vi "9203 8Ch Analog Input.vi"(1 "9203 I/O":T1={"9203 AI0"="NI 9203/AI0", "9203 AI1"="NI 9203/AI1", "9203 AI2"="NI 9203/AI2", "9203 AI3"="NI 9203/AI3", "9203 AI4"="NI 9203/AI4", "9203 AI5"="NI 9203/AI5", "9203 AI6"="NI 9203/AI6", "9203 AI7"="NI 9203/AI7"}) -> (0 "Packets":u64[](array[numeric]))   [LabVIEW 2010]
uses:
  <vilib>/eio/EIONode/EIONode.xnode
  <vilib>/rvi/eio/nirviEIOImplementation/nirviEIOImplementation.xnode
  <vilib>/rvi/eio/common/nirviEmuClasses.ctl
  <vilib>/rvi/eio/common/nirviEmuTemplateMethod_noerrors.vi
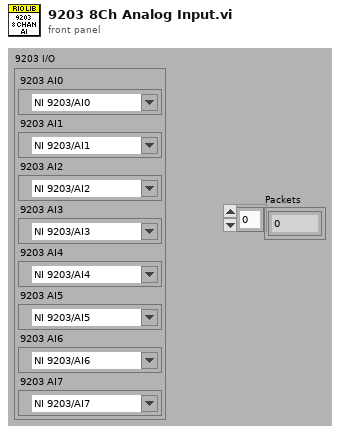
[diagram p1: front panel]
types:
  T1 = cluster{"9203 AI0":refnum<k21>, "9203 AI1":refnum<k21>, "9203 AI2":refnum<k21>, "9203 AI3":refnum<k21>, "9203 AI4":refnum<k21>, "9203 AI5":refnum<k21>, "9203 AI6":refnum<k21>, "9203 AI7":refnum<k21>}
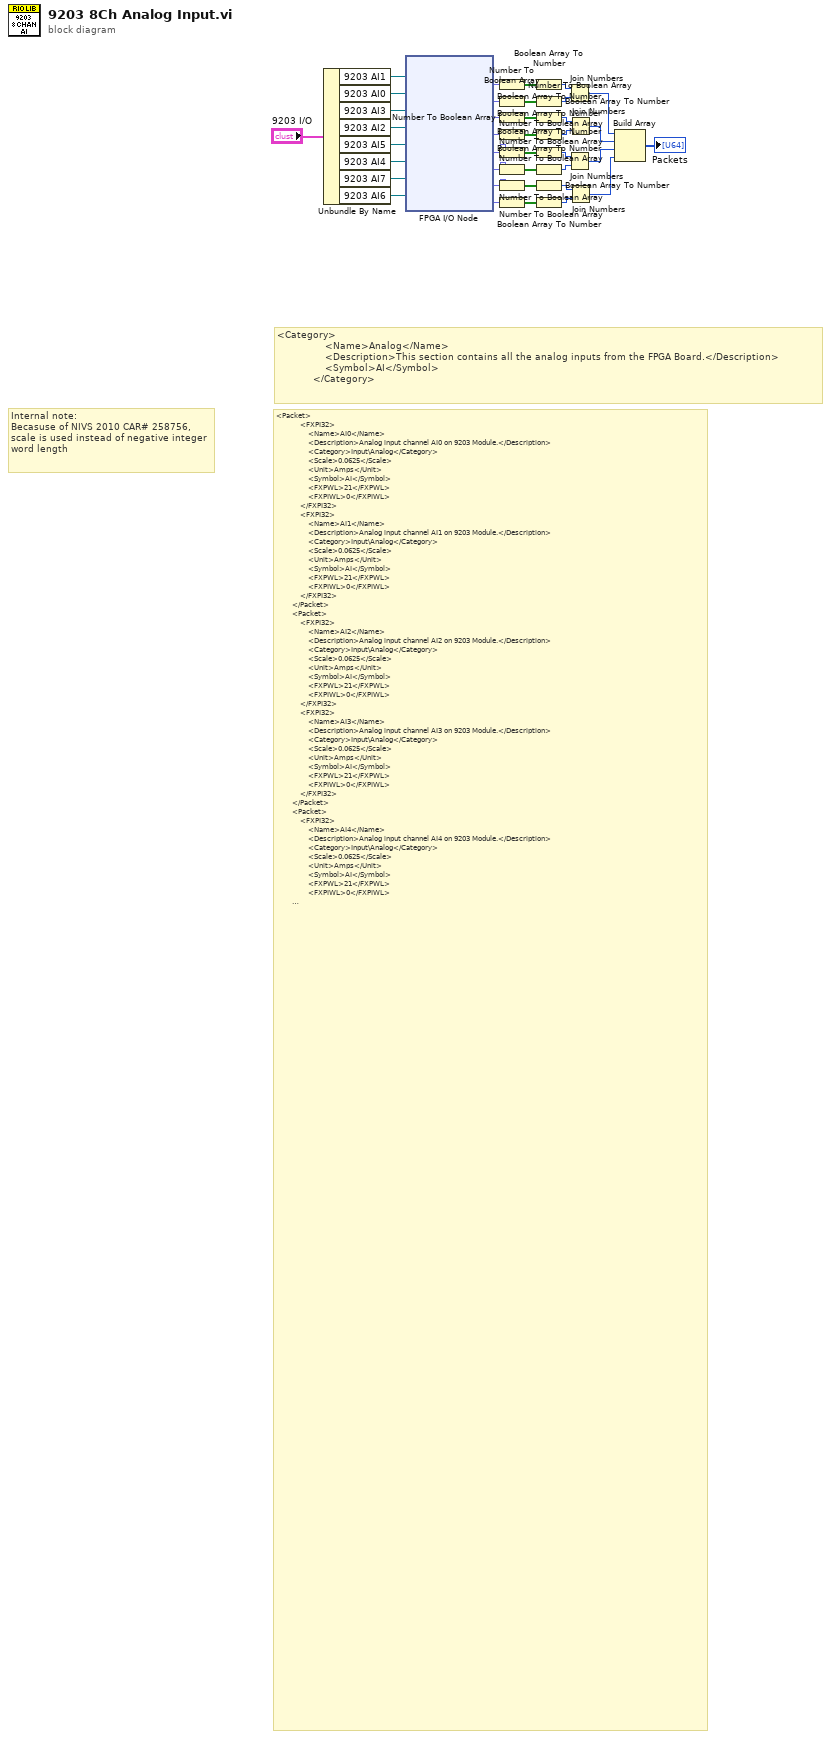
[diagram p0: block diagram]
diagram:
  # "Internal note:\nBecasuse of NIVS 2010 CAR# 258756, scale is used instead of negative integer word length"
  # "<Category>\n                <Name>Analog</Name>\n                <Description>This section contains all the analog inputs from the FPGA Board.</Description>\n                <Symbol>AI</Symbol>\n            </Category>"
  # "<Packet>\n            <FXPI32>\n                <Name>AI0</Name>\n                <Description>Analog input channel AI0 on 9203 Module.</Description>\n                <Category>Input\\Analog</Category>\n                <Scale>0.0625</Scale>\n                <Unit>Amps</Unit>\n                <Symbol>AI</Symbol>\n                <FXPWL>21</FXPWL>\n                <FXPIWL>0</FXPIWL>\n            </FXPI32>\n            <FXPI32>\n                <Name>AI1</Name>\n                <Description>Analog input channel AI1 on 9203 Module.</Description>\n                <Category>Input\\Analog</Category>\n                <Scale>0.0625</Scale>\n                <Unit>Amps</Unit>\n                <Symbol>AI</Symbol>\n                <FXPWL>21</FXPWL>\n                <FXPIWL>0</FXPIWL>\n            </FXPI32>\n        </Packet>\n        <Packet>\n            <FXPI32>\n                <Name>AI2</Name>\n                <Description>Analog input channel AI2 on 9203 Module.</Description>\n                <Category>Input\\Analog</Category>\n                <Scale>0.0625</Scale>\n                <Unit>Amps</Unit>\n                <Symbol>AI</Symbol>\n                <FXPWL>21</FXPWL>\n                <FXPIWL>0</FXPIWL>\n            </FXPI32>\n            <FXPI32>\n                <Name>AI3</Name>\n                <Description>Analog input channel AI3 on 9203 Module.</Description>\n                <Category>Input\\Analog</Category>\n                <Scale>0.0625</Scale>\n                <Unit>Amps</Unit>\n                <Symbol>AI</Symbol>\n                <FXPWL>21</FXPWL>\n                <FXPIWL>0</FXPIWL>\n            </FXPI32>\n        </Packet>\n        <Packet>\n            <FXPI32>\n                <Name>AI4</Name>\n                <Description>Analog input channel AI4 on 9203 Module.</Description>\n                <Category>Input\\Analog</Category>\n                <Scale>0.0625</Scale>\n                <Unit>Amps</Unit>\n                <Symbol>AI</Symbol>\n                <FXPWL>21</FXPWL>\n                <FXPIWL>0</FXPIWL>\n            </FXPI32>\n            <FXPI32>\n                <Name>AI5</Name>\n                <Description>Analog input channel AI5 on 9203 Module.</Description>\n                <Category>Input\\Analog</Category>\n                <Scale>0.0625</Scale>\n                <Unit>Amps</Unit>\n                <Symbol>AI</Symbol>\n                <FXPWL>21</FXPWL>\n                <FXPIWL>0</FXPIWL>\n            </FXPI32>\n        </Packet>\n        <Packet>\n            <FXPI32>\n                <Name>AI6</Name>\n                <Description>Analog input channel AI6 on 9203 Module.</Description>\n                <Category>Input\\Analog</Category>\n                <Scale>0.0625</Scale>\n                <Unit>Amps</Unit>\n                <Symbol>AI</Symbol>\n                <FXPWL>21</FXPWL>\n                <FXPIWL>0</FXPIWL>\n            </FXPI32>\n            <FXPI32>\n                <Name>AI7</Name>\n                <Description>Analog input channel AI7 on 9203 Module.</Description>\n                <Category>Input\\Analog</Category>\n                <Scale>0.0625</Scale>\n                <Unit>Amps</Unit>\n                <Symbol>AI</Symbol>\n                <FXPWL>21</FXPWL>\n                <FXPIWL>0</FXPIWL>\n            </FXPI32>\n        </Packet>"
  n1 = Unbundle By Name("9203 I/O") -> ("9203 AI1"=w19:refnum<k21>, "9203 AI0"=w22:refnum<k21>, "9203 AI3"=w20:refnum<k21>, "9203 AI2"=w23:refnum<k21>, "9203 AI5"=w15:refnum<k21>, "9203 AI4"=w16:refnum<k21>, "9203 AI7"=w17:refnum<k21>, "9203 AI6"=w18:refnum<k21>)
  n2 = xnode "FPGA I/O Node"("FPGA I/O In"=w19, "FPGA I/O In"=w22, "FPGA I/O In"=w20, "FPGA I/O In"=w23, "FPGA I/O In"=w15, "FPGA I/O In"=w16, "FPGA I/O In"=w17, "FPGA I/O In"=w18) -> ("I/O Item"=w29:fxp<+/-,21,-4>, "I/O Item"=w31:fxp<+/-,21,-4>, "I/O Item"=w21:fxp<+/-,21,-4>, "I/O Item"=w30:fxp<+/-,21,-4>, "I/O Item"=w3:fxp<+/-,21,-4>, "I/O Item"=w4:fxp<+/-,21,-4>, "I/O Item"=w5:fxp<+/-,21,-4>, "I/O Item"=w6:fxp<+/-,21,-4>)  [unwired: 8 out]
  n3 = Number To Boolean Array(number=w29) -> (Boolean array=w25:bool[])
  n4 = Number To Boolean Array(number=w31) -> (Boolean array=w26:bool[])
  n5 = Number To Boolean Array(number=w21) -> (Boolean array=w28:bool[])
  n6 = Number To Boolean Array(number=w30) -> (Boolean array=w27:bool[])
  n7 = Number To Boolean Array(number=w3) -> (Boolean array=w14:bool[])
  n8 = Number To Boolean Array(number=w4) -> (Boolean array=w13:bool[])
  n9 = Number To Boolean Array(number=w5) -> (Boolean array=w11:bool[])
  n10 = Number To Boolean Array(number=w6) -> (Boolean array=w12:bool[])
  n11 = Boolean Array To Number(Boolean array=w25) -> (number=w32:u32)
  n12 = Boolean Array To Number(Boolean array=w26) -> (number=w33:u32)
  n13 = Boolean Array To Number(Boolean array=w28) -> (number=w34:u32)
  n14 = Boolean Array To Number(Boolean array=w27) -> (number=w35:u32)
  n15 = Boolean Array To Number(Boolean array=w14) -> (number=w10:u32)
  n16 = Boolean Array To Number(Boolean array=w13) -> (number=w9:u32)
  n17 = Boolean Array To Number(Boolean array=w11) -> (number=w8:u32)
  n18 = Boolean Array To Number(Boolean array=w12) -> (number=w7:u32)
  n19 = Join Numbers(hi=w32, lo=w33) -> ((hi.lo)=w36:u64)
  n20 = Join Numbers(hi=w10, lo=w9) -> ((hi.lo)=w2:u64)
  n21 = Join Numbers(hi=w34, lo=w35) -> ((hi.lo)=w37:u64)
  n22 = Join Numbers(hi=w8, lo=w7) -> ((hi.lo)=w1:u64)
  n23 = Build Array(w36, w37, w2, w1) -> (→"Packets":u64[])
